vi "ID_Connection.vi"(5 "error in":errorcluster) -> (14 "Arduino Uno":refnum<visa-resource-name>, 15 "Arduino Uno":bool, 16 "Pump":refnum<visa-resource-name>, 17 "Pump":bool, 18 "Arduino Mega":refnum<visa-resource-name>, 19 "Arduino Mega":bool)   [LabVIEW 2024]
uses:
  <vilib>/Instr/_visa.llb/VISA Find Search Mode.ctl
  154e74cf-856d-46b8-b8e9-1ea27d1d26b1.vi
  62d40bb6-eb46-4c2a-b9a7-6b4029ac7ca3.vi
  <vilib>/regexp/Match Regular Expression.xnode
panel:
  out "Array 2":bool[](array[boolean])
  out "Numeric":i32
  out "Array":string[](array[string])
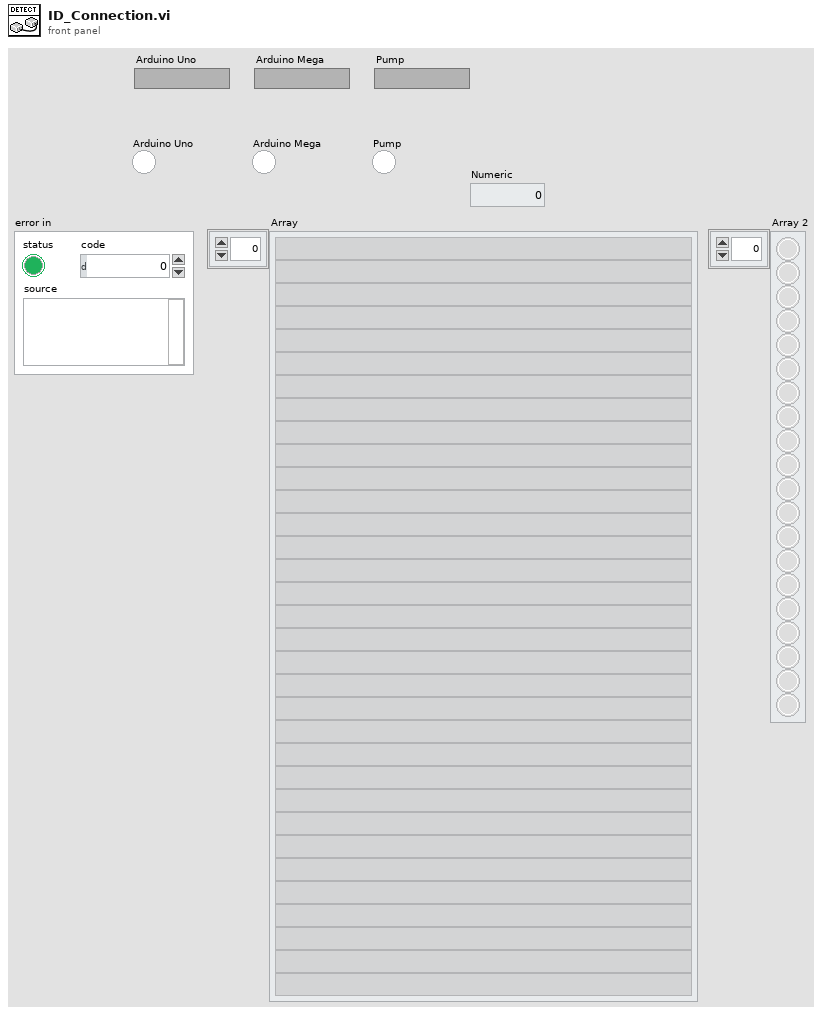
[diagram p1: front panel]
types:
  T1 = cluster{"VISA resource name":refnum<visa-resource-name>, "error out":errorcluster}
  T2 = typedef "VISA Find Search Mode.ctl" = u32
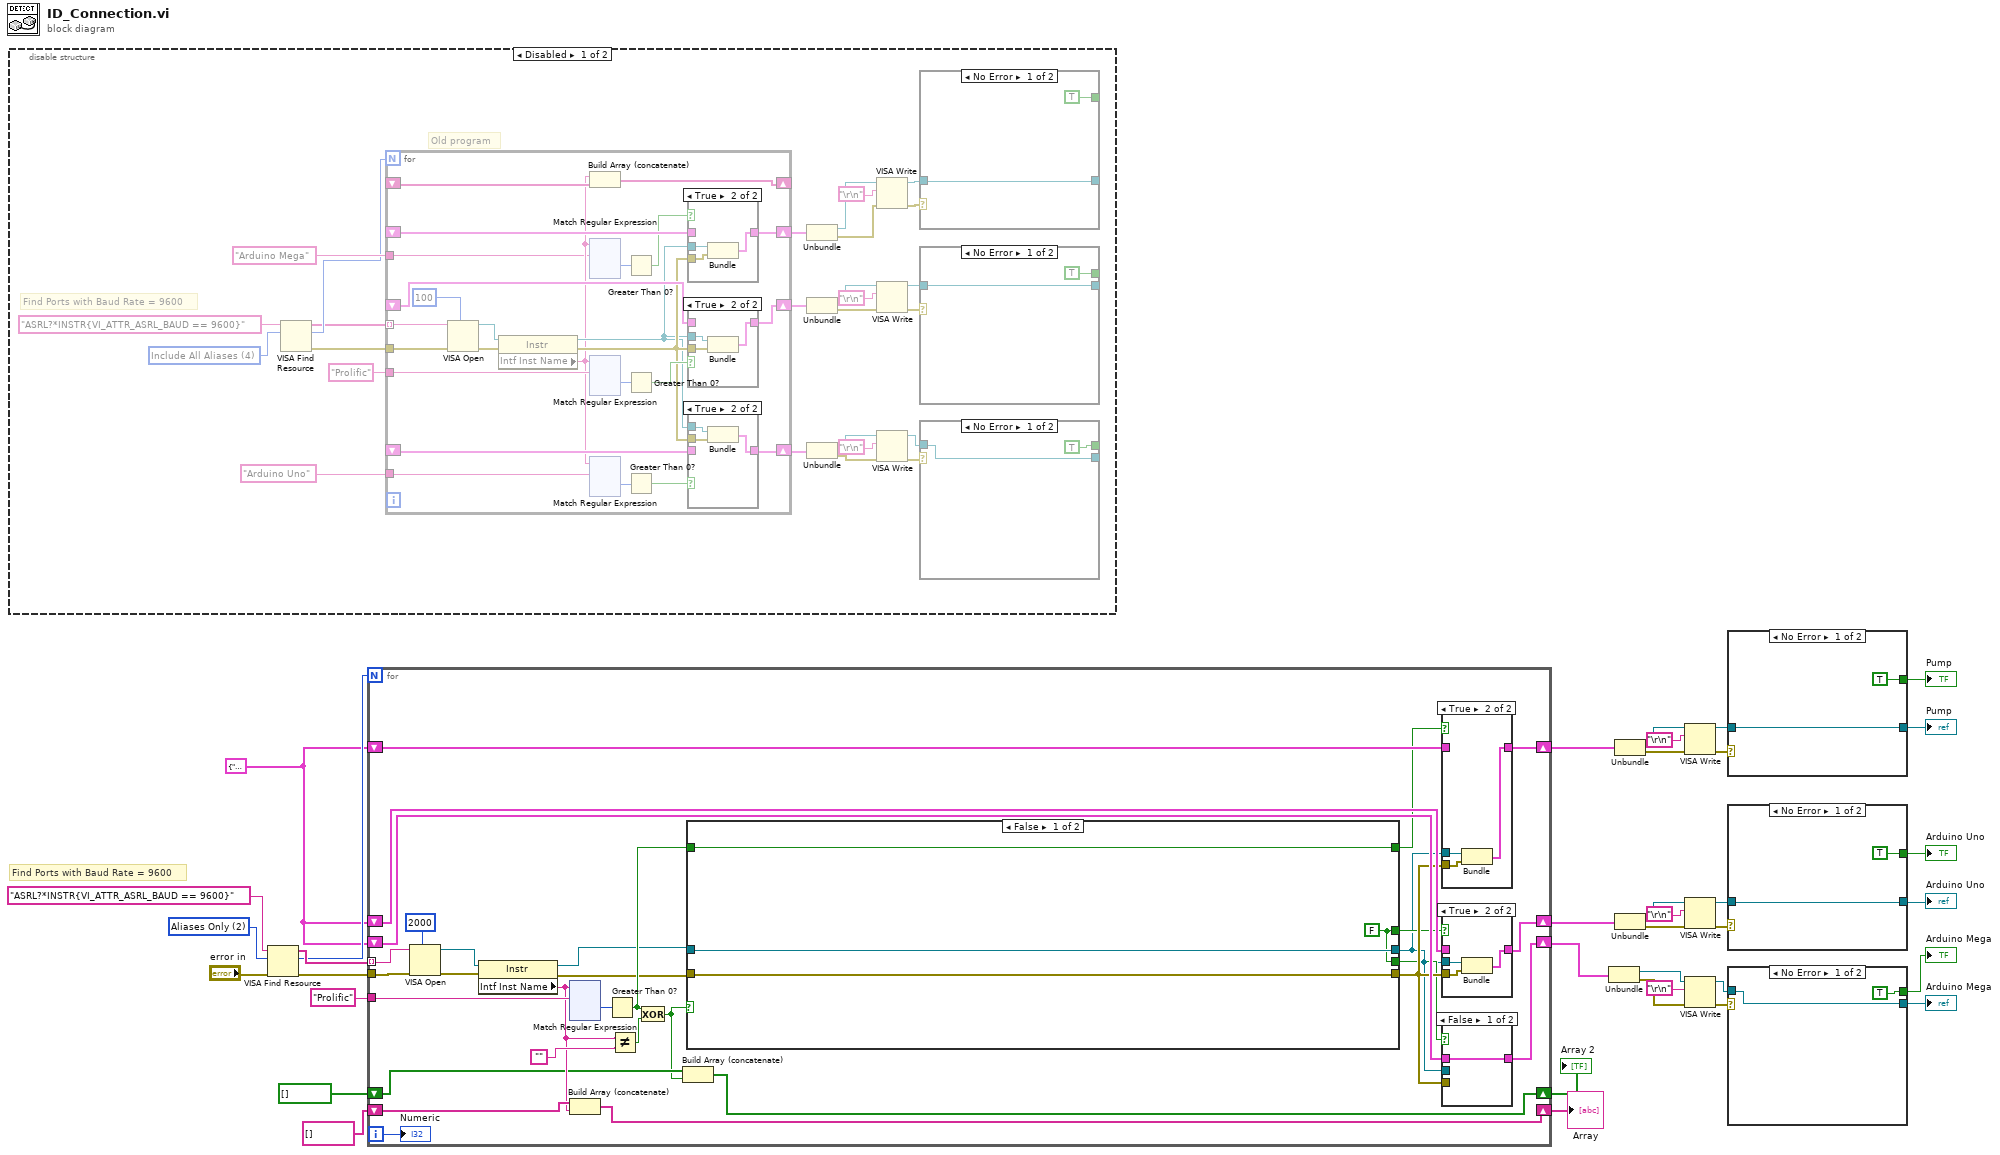
[diagram p0: block diagram]
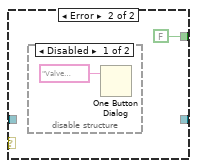
[diagram p2: hidden frame]
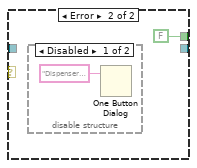
[diagram p4: hidden frame]
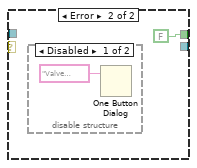
[diagram p6: hidden frame]
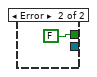
[diagram p12: hidden frame]
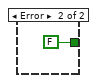
[diagram p13: hidden frame]
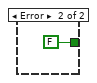
[diagram p14: hidden frame]
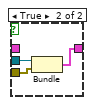
[diagram p15: hidden frame]
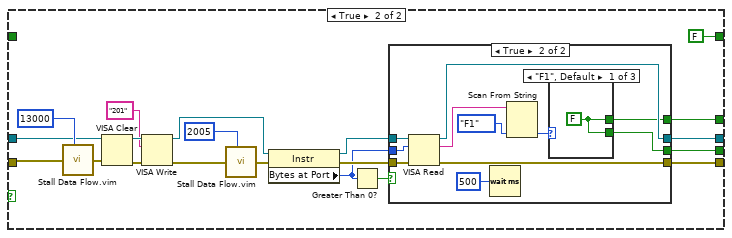
[diagram p16: hidden frame]
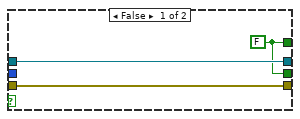
[diagram p17: hidden frame]
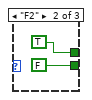
[diagram p18: hidden frame]
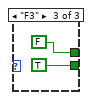
[diagram p19: hidden frame]
diagram:
  w1 = T1 {"VISA resource name"="", "error out"={"status"=FALSE, "code"=0, "source"=""}}
  w32 = T2 2 items=["Canonical Names Only"=0, "Aliases Only"=2, "Include Matching Aliases"=3, "Include All Aliases"=4] ("Search Mode")
  # "Find Ports with Baud Rate = 9600"
  n1 = disable-structure shown="Disabled" {
    frame Disabled {
      w41 = T2 4 items=["Canonical Names Only"=0, "Aliases Only"=2, "Include Matching Aliases"=3, "Include All Aliases"=4] ("Search Mode")
      # "Old program"
      # "Find Ports with Baud Rate = 9600"
      n2 = VISA Find Resource(10:w41, 11:"ASRL?*INSTR{VI_ATTR_ASRL_BAUD == 9600}" ("expression (\"?*\")")) -> (0:w40:errorcluster, 2:w51:u32, 3:w37:string[])  [unwired: 1 in]
      n3 = for {
        N: w51 -> [_]
        tunnel: w37 -> [w99] mode=indexing
        tunnel: "Arduino Uno" -> [w95]
        shift-right: [w93] -> w38
        shift-left: _ -> [w92]
        tunnel: w40 -> [w91]
        shift-right: [w90] -> w43
        shift-left: _ -> [w89]
        tunnel: "Prolific" -> [w86]
        shift-right: [w84] -> _
        shift-left: _ -> [w83]
        shift-right: [w82] -> w61
        shift-left: _ -> [w79]
        tunnel: "Arduino Mega" ("regular expression") -> [w77]
        n4 = VISA Open(timeout (0)=u32 100 ("VISA Open timeout (0)"), error in (no error)=w91, VISA resource name=w99) -> (VISA resource name=w98:refnum<visa-resource-name>, error out=w94:errorcluster)  [unwired: 2 in]
        n5 = property class="Instr"(reference=w98, error in=w94) -> (reference out=w80:refnum<visa-resource-name>, error out=w81:errorcluster, "Intf Inst Name"=w78:string)
        n6 = Build Array (concatenate)(w78, w83) -> (w84:string[])
        n7 = xnode "Match Regular Expression"("input string"=w78, "regular expression"=w77) -> ("offset past match"=w75:i32)  [unwired: 4 in, 4 out]
        n8 = xnode "Match Regular Expression"("input string"=w78, "regular expression"=w86) -> ("offset past match"=w88:i32)  [unwired: 4 in, 4 out]
        n9 = xnode "Match Regular Expression"("input string"=w78, "regular expression"=w95) -> ("offset past match"=w97:i32)  [unwired: 4 in, 4 out]
        n10 = Greater Than 0?(x=w75) -> (x > 0?=w76:bool)
        n11 = Greater Than 0?(x=w88) -> (x > 0?=w87:bool)
        n12 = Greater Than 0?(x=w97) -> (x > 0?=w96:bool)
        n13 = case shown="True" w76 {
          tunnel: w80 -> [_ w220]
          tunnel: w81 -> [_ w219]
          tunnel: [w217 w218] -> w82
          tunnel: w79 -> [w217 _]
          frame False {
          }
          frame True {
            n14 = Bundle("VISA resource name"=w220, "error out"=w219) -> (w218:T1)  [unwired: 1 in]
          }
        }
        n15 = case shown="True" w87 {
          tunnel: w80 -> [_ w341]
          tunnel: w81 -> [_ w340]
          tunnel: [w338 w339] -> w90
          tunnel: w89 -> [w338 _]
          frame False {
          }
          frame True {
            n16 = Bundle("VISA resource name"=w341, "error out"=w340) -> (w339:T1)  [unwired: 1 in]
          }
        }
        n17 = case shown="True" w96 {
          tunnel: w80 -> [_ w345]
          tunnel: w81 -> [_ w344]
          tunnel: [w342 w343] -> w93
          tunnel: w92 -> [w342 _]
          frame False {
          }
          frame True {
            n18 = Bundle("VISA resource name"=w345, "error out"=w344) -> (w343:T1)  [unwired: 1 in]
          }
        }
      }
      n19 = Unbundle(w61) -> ("VISA resource name"=w57:refnum<visa-resource-name>, "error out"=w56:errorcluster)
      n20 = Unbundle(w43) -> ("VISA resource name"=w55:refnum<visa-resource-name>, "error out"=w54:errorcluster)
      n21 = Unbundle(w38) -> ("VISA resource name"=w52:refnum<visa-resource-name>, "error out"=w53:errorcluster)
      n22 = VISA Write(VISA resource name=w57, write buffer="\r\n", error in (no error)=w56) -> (VISA resource name out=w60:refnum<visa-resource-name>, error out=w59:errorcluster)  [unwired: 1 out]
      n23 = VISA Write(VISA resource name=w55, write buffer="\r\n", error in (no error)=w54) -> (VISA resource name out=w47:refnum<visa-resource-name>, error out=w46:errorcluster)  [unwired: 1 out]
      n24 = VISA Write(VISA resource name=w52, write buffer="\r\n", error in (no error)=w53) -> (VISA resource name out=w44:refnum<visa-resource-name>, error out=w45:errorcluster)  [unwired: 1 out]
      n25 = case shown="No Error" w59 {
        tunnel: [TRUE FALSE] -> _
        tunnel: w60 -> [w63 _]
        tunnel: [w63 _] -> _
        frame No Error {
        }
        frame Error {
          n26 = disable-structure shown="Disabled" {
            frame Disabled {
              n27 = One Button Dialog(message="Valve Connection Error!") -> ()  [unwired: 1 in, 1 out]
            }
            frame Enabled {
            }
          }
        }
      }
      n28 = case shown="No Error" w46 {
        tunnel: [w68 _] -> _
        tunnel: w47 -> [w68 _]
        tunnel: [TRUE FALSE] -> _
        frame No Error {
        }
        frame Error {
          n29 = disable-structure shown="Disabled" {
            frame Disabled {
              n30 = One Button Dialog(message="Dispenser Connection Error!") -> ()  [unwired: 1 in, 1 out]
            }
            frame Enabled {
            }
          }
        }
      }
      n31 = case shown="No Error" w45 {
        tunnel: [TRUE FALSE] -> _
        tunnel: w44 -> [w71 _]
        tunnel: [w71 _] -> _
        frame No Error {
        }
        frame Error {
          n32 = disable-structure shown="Disabled" {
            frame Disabled {
              n33 = One Button Dialog(message="Valve Connection Error!") -> ()  [unwired: 1 in, 1 out]
            }
            frame Enabled {
            }
          }
        }
      }
    }
    frame Enabled {
    }
  }
  n34 = VISA Find Resource(8:"error in", 10:w32, 11:"ASRL?*INSTR{VI_ATTR_ASRL_BAUD == 9600}" ("expression (\"?*\")")) -> (0:w34:errorcluster, 2:w18:u32, 3:w36:string[])
  n35 = for {
    N: w18 -> [_]
    tunnel: w36 -> [w492] mode=indexing
    shift-right: [w490] -> w35
    shift-left: w1 -> [w489]
    tunnel: w34 -> [w488]
    shift-right: [w487] -> w30
    shift-left: w1 -> [w486]
    tunnel: "Prolific" -> [w484]
    shift-right: [w482] -> w17
    shift-left: string[] [] -> [w467]
    shift-right: [w481] -> w5
    shift-left: w1 -> [w480]
    shift-right: [w473] -> w4
    shift-left: bool[] [] -> [w465]
    i -> [w474]
    n36 = VISA Open(timeout (0)=u32 2000 ("VISA Open timeout (0)"), error in (no error)=w488, VISA resource name=w492) -> (VISA resource name=w491:refnum<visa-resource-name>, error out=w469:errorcluster)  [unwired: 2 in]
    n37 = property class="Instr"(reference=w491, error in=w469) -> (reference out=w468:refnum<visa-resource-name>, error out=w463:errorcluster, "Intf Inst Name"=w466:string)
    n38 = xnode "Match Regular Expression"("input string"=w466, "regular expression"=w484) -> ("offset past match"=w485:i32)  [unwired: 4 in, 4 out]
    n39 = Build Array (concatenate)(w467, w466) -> (w482:string[])
    n40 = Greater Than 0?(x=w485) -> (x > 0?=w470:bool)
    n41 = Not Equal?(x=w466, y="") -> (x != y?=w471:bool)
    n42 = Exclusive Or(1:w471, 2:w470) -> (0:w464:bool)
    n43 = Build Array (concatenate)(w465, w464) -> (w473:bool[])
    n44 = case shown="False" w464 {
      tunnel: w468 -> [w500 w502]
      tunnel: w463 -> [w499 w501]
      tunnel: [w500 w513] -> w476
      tunnel: [w499 w512] -> w479
      tunnel: [w498 w510] -> w478
      tunnel: [w498 w511] -> w477
      tunnel: [w497 FALSE] -> w475
      tunnel: w470 -> [w497 _]
      frame False {
        w498 = FALSE
      }
      frame True {
        n45 = call "Stall Data Flow.vim"("value in"=w501, "milliseconds to wait"=u32 13000) -> ("value out"=w504:errorcluster)  [unwired: 1 out]
        n46 = VISA Clear(VISA resource name=w502, error in (no error)=w504) -> (VISA resource name out=w519:refnum<visa-resource-name>, error out=w520:errorcluster)
        n47 = VISA Write(VISA resource name=w519, write buffer="201", error in (no error)=w520) -> (VISA resource name out=w517:refnum<visa-resource-name>, error out=w508:errorcluster)  [unwired: 1 out]
        n48 = call "Stall Data Flow.vim"("value in"=w508, "milliseconds to wait"=u32 2005) -> ("value out"=w507:errorcluster)  [unwired: 1 out]
        n49 = property class="Instr"(reference=w517, error in=w507) -> (reference out=w515:refnum<visa-resource-name>, error out=w514:errorcluster, "Bytes at Port"=w509:u32)
        n50 = Greater Than 0?(x=w509) -> (x > 0?=w516:bool)
        n51 = case shown="True" w516 {
          tunnel: w515 -> [w523 w534]
          tunnel: w514 -> [w522 w533]
          tunnel: [w523 w532] -> w513
          tunnel: [w522 w531] -> w512
          tunnel: [w521 w529] -> w511
          tunnel: [w521 w530] -> w510
          tunnel: w509 -> [_ w525]
          frame False {
            w521 = FALSE
          }
          frame True {
            n52 = VISA Read(VISA resource name=w534, byte count=w525, error in (no error)=w533) -> (VISA resource name out=w532:refnum<visa-resource-name>, read buffer=w528:string, error out=w531:errorcluster)  [unwired: 1 out]
            n53 = Wait (ms)(milliseconds to wait=u32 500) -> ()  [unwired: 1 out]
            n54 = Scan From String(input string=w528, default 1=enum16{"F1", "F2", "F3"}."F1") -> (output 1=w526:enum16{"F1", "F2", "F3"})  [unwired: 3 in, 3 out]
            n55 = case shown="\"F1\", Default" w526 {
              tunnel: [w535 FALSE TRUE] -> w530
              tunnel: [w535 TRUE FALSE] -> w529
              frame "F1", Default {
                w535 = FALSE
              }
              frame "F2" {
              }
              frame "F3" {
              }
            }
          }
        }
      }
    }
    n56 = case shown="True" w475 {
      tunnel: w476 -> [_ w660]
      tunnel: w479 -> [_ w659]
      tunnel: [w657 w658] -> w487
      tunnel: w486 -> [w657 _]
      frame False {
      }
      frame True {
        n57 = Bundle("VISA resource name"=w660, "error out"=w659) -> (w658:T1)  [unwired: 1 in]
      }
    }
    n58 = case shown="True" w477 {
      tunnel: w476 -> [_ w664]
      tunnel: w479 -> [_ w663]
      tunnel: [w661 w662] -> w490
      tunnel: w489 -> [w661 _]
      frame False {
      }
      frame True {
        n59 = Bundle("VISA resource name"=w664, "error out"=w663) -> (w662:T1)  [unwired: 1 in]
      }
    }
    n60 = case shown="False" w478 {
      tunnel: w476 -> [_ w496]
      tunnel: w479 -> [_ w495]
      tunnel: [w493 w494] -> w481
      tunnel: w480 -> [w493 _]
      frame False {
      }
      frame True {
        n61 = Bundle("VISA resource name"=w496, "error out"=w495) -> (w494:T1)  [unwired: 1 in]
      }
    }
    "Numeric" <- w474
  }
  "Array" <- w17
  "Array 2" <- w4
  n62 = Unbundle(w5) -> ("VISA resource name"=w7:refnum<visa-resource-name>, "error out"=w6:errorcluster)
  n63 = Unbundle(w30) -> ("VISA resource name"=w13:refnum<visa-resource-name>, "error out"=w14:errorcluster)
  n64 = Unbundle(w35) -> ("VISA resource name"=w16:refnum<visa-resource-name>, "error out"=w15:errorcluster)
  n65 = VISA Write(VISA resource name=w13, write buffer="\r\n", error in (no error)=w14) -> (VISA resource name out=w23:refnum<visa-resource-name>, error out=w25:errorcluster)  [unwired: 1 out]
  n66 = VISA Write(VISA resource name=w16, write buffer="\r\n", error in (no error)=w15) -> (VISA resource name out=w29:refnum<visa-resource-name>, error out=w28:errorcluster)  [unwired: 1 out]
  n67 = VISA Write(VISA resource name=w7, write buffer="\r\n", error in (no error)=w6) -> (VISA resource name out=w8:refnum<visa-resource-name>, error out=w9:errorcluster)  [unwired: 1 out]
  n68 = case shown="No Error" w25 {
    tunnel: [w666 _] -> w24
    tunnel: w23 -> [w666 _]
    tunnel: [TRUE FALSE] -> w22
    frame No Error {
    }
    frame Error {
    }
  }
  "Pump" <- w24
  "Pump" <- w22
  n69 = case shown="No Error" w28 {
    tunnel: [TRUE FALSE] -> w26
    tunnel: w29 -> [w668 _]
    tunnel: [w668 _] -> w27
    frame No Error {
    }
    frame Error {
    }
  }
  "Arduino Uno" <- w27
  "Arduino Uno" <- w26
  n70 = case shown="No Error" w9 {
    tunnel: [TRUE FALSE] -> w11
    tunnel: w8 -> [w671 _]
    tunnel: [w671 _] -> w10
    frame No Error {
    }
    frame Error {
    }
  }
  "Arduino Mega" <- w10
  "Arduino Mega" <- w11
